vi "Periodic Tasks.vi"(8 "error in":errorcluster) -> ()   [LabVIEW 2020]
doc: "This VI runs in parallel to other tasks. It can contain as many user-defined periodic loops as you need. These can carry out PID or other sorts of timed response."
uses:
  <vilib>/Rock Robotics/WPI/ThirdParty/Sensors/navX/_Processing Loop/FRIC_navX_Internal_SPI_ProcessingLoop.vi
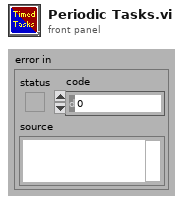
[diagram p1: front panel]
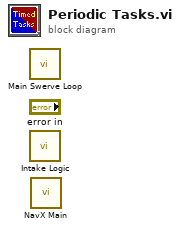
[diagram p0: block diagram]
diagram:
  n1 = call "Main Swerve Loop.vi"() -> ()  [unwired: 12 in]
  n2 = call "Intake Logic.vi"() -> ()  [unwired: 12 in]
  n3 = call-poly <vilib>:"NavX Main.vi"() -> ()  [unwired: 12 in]
